vi "Partial Derivatives of f(x1,x2).vi"(5 "Variables":string[](array[string])=["x1", "x2"], 6 "formula":string, 7 "derivative":u16(ring) items=["first variable", "second variable"], 8 "number of points":u32=25, 9 "End":dbl[](array[numeric])=[1.0, 1.0] format="%.2f", 10 "Start":dbl[](array[numeric])=[0.0, 0.0] format="%.2f") -> (0 "error":i32, 1 "ticks":u32, 2 "Partial derivative of f(x1,x2)":dbl[][](array[numeric]) format="%.2f", 3 "X2 Values":dbl[](array[numeric]) format="%.2f", 4 "X1 Values":dbl[](array[numeric]) format="%.2f")   [LabVIEW 2017, in "NI_Gmath.lvlib"]
doc: "Calculates a 2D array of the partial derivatives of a function of two independent variables."
uses:
  NI_Gmath.lvlib
panel:
  # "Example:\n\n number of points: 25\n Start: 0.0 and 0.0\n End: 1.0 and 1.0\n derivative: first variable\n Variables: x1 and x2 \n formula: 7*sin(x1)^2+cos(3*x2)^2"
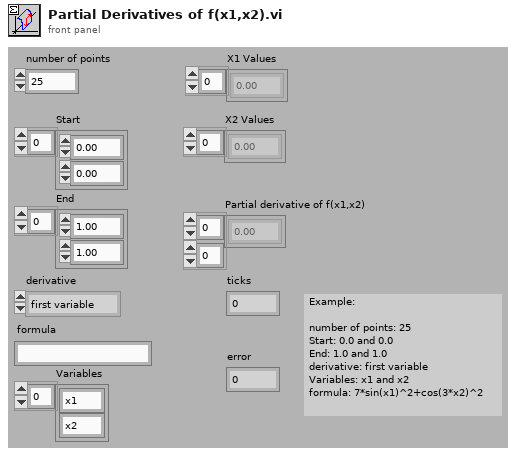
[diagram p1: front panel]
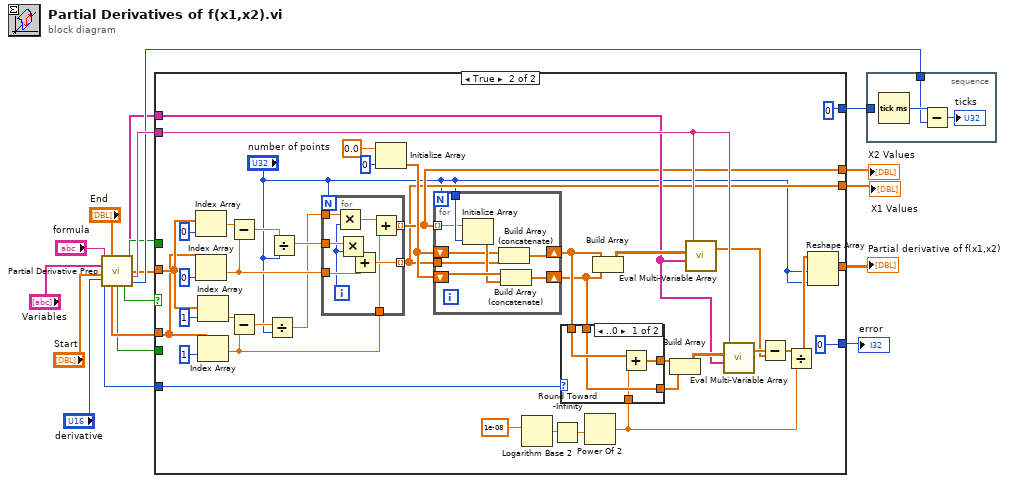
[diagram p0: block diagram]
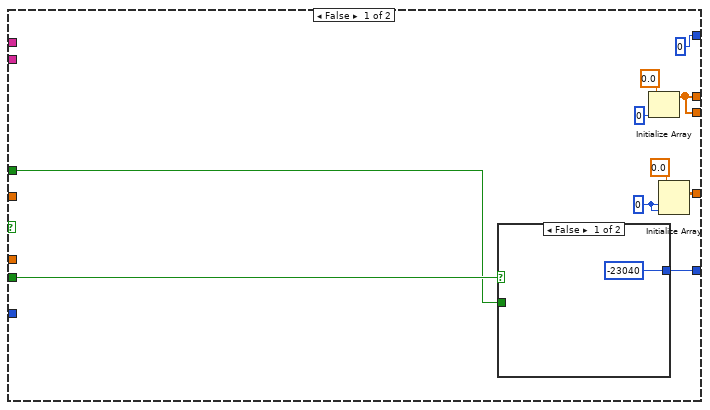
[diagram p2: hidden frame]
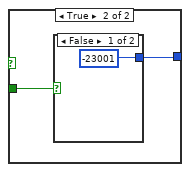
[diagram p3: hidden frame]
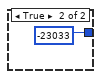
[diagram p4: hidden frame]
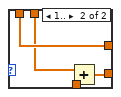
[diagram p5: hidden frame]
diagram:
  n1 = call "Partial Derivative Prep.vi"("formula"="formula", "End"="End", "Variables"="Variables", "Start"="Start", "derivative"="derivative") -> ("Variables"=w6:string[], "formula"=w18:string, "End"=w14:dbl[], 10:w17:u32, "derivative"=w12:u16, "Start"=w13:dbl[], "specific error 2"=w11:bool, "error (general)"=w5:bool, "specific error 1"=w9:bool)  [unwired: 2 in]
  n2 = case shown="True" w5 {
    tunnel: [0 0] -> w19
    tunnel: w18 -> [_ w50]
    tunnel: w6 -> [_ w42]
    tunnel: [w26 w58] -> w16
    tunnel: w14 -> [_ w41]
    tunnel: w13 -> [_ w40]
    tunnel: w12 -> [_ w39]
    tunnel: w11 -> [w25 _]
    tunnel: [w24 0] -> w10
    tunnel: w9 -> [w23 _]
    tunnel: [w20 w37] -> w8
    tunnel: [w20 w36] -> w7
    frame False {
      w27 = 0
      n3 = case shown="False" w25 {
        tunnel: [-23040 w32] -> w24
        tunnel: w23 -> [_ w31]
        frame False {
        }
        frame True {
          n4 = case shown="False" w31 {
            tunnel: [-23001 -23033] -> w32
            frame False {
            }
            frame True {
            }
          }
        }
      }
      n5 = Initialize Array(0.0, 0) -> (w20:dbl[])
      n6 = Initialize Array(0.0, w27, w27) -> (w26:dbl[][])
    }
    frame True {
      n7 = Index Array(array=w41, index=0) -> (element=w70:dbl)
      n8 = Index Array(array=w40, index=0) -> (element=w71:dbl)
      n9 = Index Array(array=w41, index=1) -> (element=w72:dbl)
      n10 = Index Array(array=w40, index=1) -> (element=w73:dbl)
      n11 = Subtract(x=w70, y=w71) -> (x-y=w59:dbl)
      n12 = Subtract(x=w72, y=w73) -> (x-y=w63:dbl)
      n13 = Divide(x=w63, y="number of points") -> (x/y=w64:dbl)
      n14 = Divide(x=w59, y="number of points") -> (x/y=w65:dbl)
      n15 = for {
        N: "number of points" -> [_]
        tunnel: w65 -> [w91]
        tunnel: w71 -> [w89]
        tunnel: [w88] -> w36 mode=indexing
        tunnel: w64 -> [w87]
        tunnel: w73 -> [w84]
        tunnel: [w83] -> w37 mode=indexing
        i -> [w86]
        n16 = Multiply(x=w87, y=w86) -> (x*y=w85:dbl)
        n17 = Multiply(x=w91, y=w86) -> (x*y=w90:dbl)
        n18 = Add(x=w90, y=w89) -> (x+y=w88:dbl)
        n19 = Add(x=w85, y=w84) -> (x+y=w83:dbl)
      }
      n20 = Initialize Array(0.0, 0) -> (w62:dbl[])
      n21 = for {
        N: "number of points" -> [_]
        tunnel: "number of points" -> [w99]
        tunnel: w37 -> [w98] mode=indexing
        shift-right: [w96] -> w51
        shift-left: w62 -> [w97]
        shift-right: [w94] -> w52
        shift-left: w62 -> [w93]
        tunnel: w36 -> [w92]
        n22 = Initialize Array(w98, w99) -> (w95:dbl[])
        n23 = Build Array (concatenate)(w93, w92) -> (w94:dbl[])
        n24 = Build Array (concatenate)(w97, w95) -> (w96:dbl[])
      }
      n25 = Logarithm Base 2(1:1e-08) -> (0:w57:dbl)
      n26 = Round Toward -Infinity(1:w57) -> (0:w56:dbl)
      n27 = Power Of 2(x=w56) -> (2^x=w46:dbl)
      n28 = case shown="..0" w39 {
        tunnel: w52 -> [w78 w82]
        tunnel: [w77 w82] -> w55
        tunnel: w51 -> [w76 w81]
        tunnel: [w76 w79] -> w54
        tunnel: w46 -> [w75 w80]
        frame ..0 {
          n29 = Add(x=w78, y=w75) -> (x+y=w77:dbl[])
        }
        frame 1.. {
          n30 = Add(x=w81, y=w80) -> (x+y=w79:dbl[])
        }
      }
      n31 = Build Array(w52, w51) -> (w44:dbl[][])
      n32 = Build Array(w55, w54) -> (w43:dbl[][])
      n33 = call "Eval Multi-Variable Array.vi"("Variables"=w42, "X Values"=w44, "formula"=w50) -> ("Y Values"=w47:dbl[])  [unwired: 1 in, 1 out]
      n34 = call "Eval Multi-Variable Array.vi"("Variables"=w42, "X Values"=w43, "formula"=w50) -> ("Y Values"=w48:dbl[])  [unwired: 1 in, 1 out]
      n35 = Subtract(x=w48, y=w47) -> (x-y=w49:dbl[])
      n36 = Divide(x=w49, y=w46) -> (x/y=w45:dbl[])
      n37 = Reshape Array(w45, "number of points", "number of points") -> (w58:dbl[][])
    }
  }
  "Partial derivative of f(x1,x2)" <- w16
  "error" <- w10
  "X2 Values" <- w8
  "X1 Values" <- w7
  n38 = stacked-sequence {
    tunnel: w19 -> [_]
    tunnel: w17 -> [w100]
    frame #0 {
      n39 = Tick Count (ms)() -> (millisecond timer value=w102:u32)
      n40 = Subtract(x=w102, y=w100) -> (x-y=→"ticks":u32)
    }
  }
